vi "Calibrate Gyro.vi"   [LabVIEW 2013]
uses:
  <vilib>/rvi/interface/nirviOpenFPGA/nirviOpenFPGA.xnode
  <vilib>/rvi/interface/nirviReadWriteControl/nirviReadWriteControl.xnode
  <vilib>/rvi/interface/Simulation/niFpgaSimulationCallBeginRW.vi
  <vilib>/rvi/errors/niLvFpgaAdjustHostInterfaceError.vi
  <vilib>/rvi/interface/nirviCloseFPGA/nirviCloseFPGA.xnode
  FPGA/Sensor Library/FPGA.vi
  <vilib>/FPGAPlugInAG/Dynamic/niLvFpga_Close_Dynamic.vi
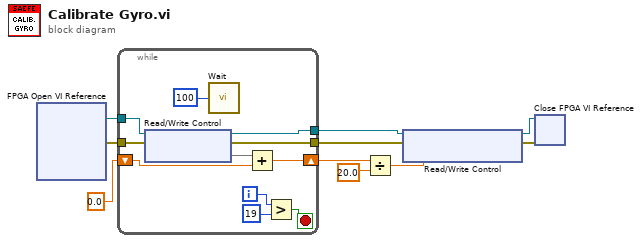
[diagram p0: block diagram]
diagram:
  n1 = xnode "FPGA Open VI Reference"() -> ("FPGA VI Reference Out"=w10:refnum<k20>, "error out"=w5:errorcluster)  [unwired: 2 in]
  n2 = while {
    tunnel: w10 -> [w17]
    shift-right: [w15] -> w8
    shift-left: 0.0 -> [w14]
    tunnel: [w13] -> w6
    tunnel: w5 -> [w12]
    tunnel: [w11] -> w4
    i -> [w19]
    stop <- w18 stop-if-true
    n3 = xnode "Read/Write Control"("FPGA VI Reference In"=w17, "error in"=w12) -> ("FPGA VI Reference Out"=w13:refnum<k20>, "error out"=w11:errorcluster, "Gyro Voltage"=w16)
    n4 = call "Wait"("Count(mSec)"=u32 100) -> ()  [unwired: 1 out]
    n5 = Add(x=w16, y=w14) -> (x+y=w15:dbl)
    n6 = Greater?(x=w19, y=19) -> (0:w18:bool)
  }
  n7 = Divide(x=w8, y=20.0) -> (x/y=w3:dbl)
  n8 = xnode "Read/Write Control"("FPGA VI Reference In"=w6, "error in"=w4, "Calibration Voltage"=w3) -> ("FPGA VI Reference Out"=w2:refnum<k20>, "error out"=w1:errorcluster)
  n9 = xnode "Close FPGA VI Reference"("FPGA VI Reference In"=w2, "error in"=w1) -> ()  [unwired: 1 out]
